vi "Move Servo_1.vi"(0 "NXT":T2={"Hardware"="NXT", "Flattened String"=""}, 2 "Servo Position 1":u8=10, 12 "Servo":cluster{"Servo":T1, "Address":i16}={"Servo"=enum."Servo", "Address"=-1}, 14 "Sync (None)":u8(ring) items=["No Sync"=0, "Slow (15)"=15, "Medium (8)"=8, "Fast (1)"=1]) -> (20 "NXT":T2={"Hardware"="NXT", "Flattened String"=""})   [LabVIEW 2010, in "4134Outputs.lvlib"]
uses:
  4134Outputs.lvlib
  <vilib>/NXT/Subs/LVHSConnector.ctl
  <vilib>/NXT/Subs/MotorXNode.Servo Type.ctl
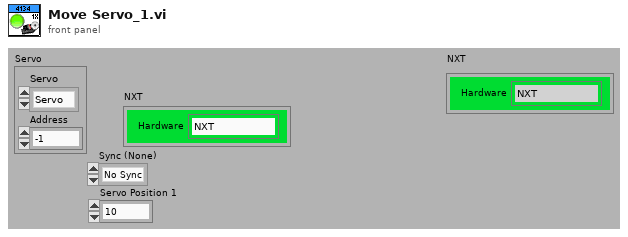
[diagram p1: front panel]
types:
  T1 = typedef "MotorXNode.Servo Type.ctl" = enum16{"Servo"}
  T2 = typedef "LVHSConnector.ctl" = cluster{"Hardware":string, "Flattened String":string}
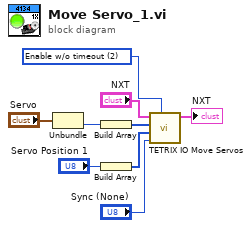
[diagram p0: block diagram]
diagram:
  w9 = u16 2 items=["Disable", "Enable w/timeout", "Enable w/o timeout"] ("Servo State (Enable w/o timeout)")
  n1 = Unbundle("Servo") -> ("Address"=w6:i16)  [unwired: 1 out]
  n2 = Build Array(w6) -> (w5:i16[])
  n3 = Build Array("Servo Position 1") -> (w4:u8[])
  n4 = call <vilib>:"TETRIX IO Move Servos.vi"("Servo State (Enable w/o timeout)"=w9, "Update Interval (0)"="Sync (None)", "Servo Positions"=w4, "Servos"=w5, "NXT"="NXT") -> ("NXT"=→"NXT":T2)  [unwired: 6 in]
